vi "get_state.vi"(8 "error in (no error)":errorcluster, 11 "DAQmxDigitalOut.lvclass in":refnum<class "DigitalOutDL110325DAQmx.lvclass">) -> (0 "error out":errorcluster, 2 "state":bool, 3 "DAQmxDigitalOut.lvclass out":refnum<class "DigitalOutDL110325DAQmx.lvclass">)   [LabVIEW 2010, in "DigitalOutDL110325DAQmx.lvclass"]
uses:
  DigitalOutDL110325DAQmx.lvclass
  DigitalOutDL110325DAQmx.lvclass/DigitalOutDL110325DAQmx.ctl
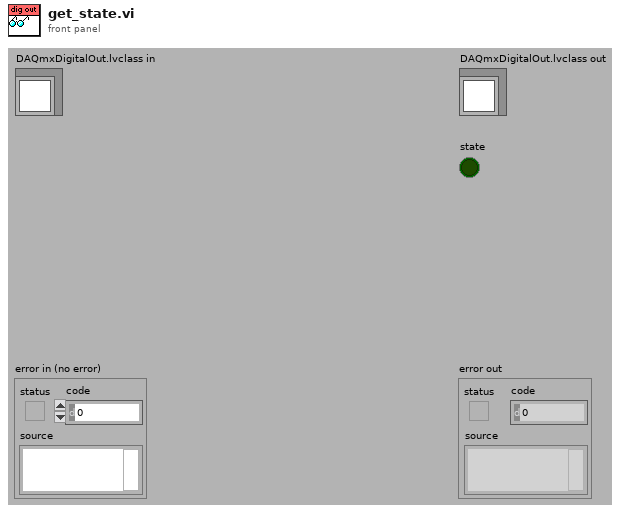
[diagram p1: front panel]
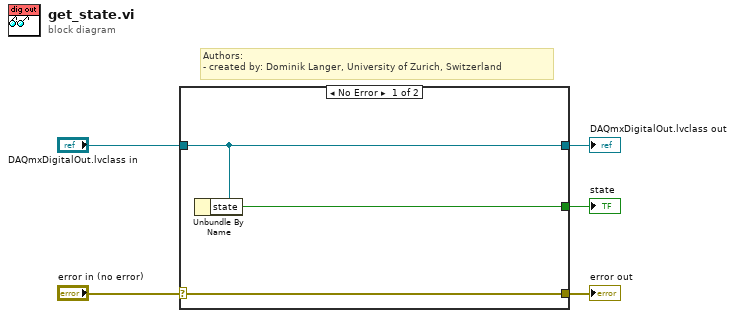
[diagram p0: block diagram]
diagram:
  # "Authors: \n- created by: Dominik Langer, University of Zurich, Switzerland"
  n1 = case shown="No Error" "error in (no error)" {
    selector: "error in (no error)" -> [w8 w9]
    tunnel: [w8 w9] -> w4
    tunnel: [w7 w10] -> w2
    tunnel: "DAQmxDigitalOut.lvclass in" -> [w7 w10]
    tunnel: [w6 _] -> w1
    frame No Error {
      n2 = Unbundle By Name(w7) -> ("state"=w6:bool)
    }
    frame Error {
    }
  }
  "error out" <- w4
  "DAQmxDigitalOut.lvclass out" <- w2
  "state" <- w1
